vi "Checkers File Load.vi"   [LabVIEW 2016]
uses:
  Game Info Global Variable.vi
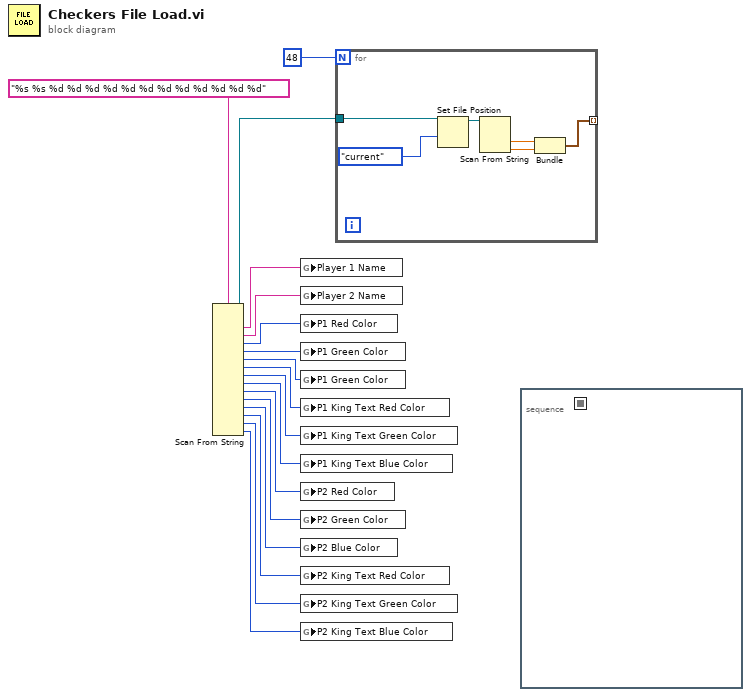
[diagram p0: block diagram]
diagram:
  n1 = Scan From String("%s %s %d %d %d %d %d %d %d %d %d %d %d %d" ("format string")) -> (w16:refnum<file>, output 1=w14:string, output 2=w13:string, output 3=w12:i32, output 4=w11:i32, output 5=w10:i32, output 6=w9:i32, output 7=w8:i32, output 8=w7:i32, output 9=w6:i32, output 10=w5:i32, output 11=w4:i32, output 12=w3:i32, output 13=w2:i32, output 14=w1:i32)  [unwired: 16 in, 1 out]
  n2 = global write "Game Info Global Variable.vi" "Player 1 Name"(w14) -> ()
  n3 = global write "Game Info Global Variable.vi" "Player 2 Name"(w13) -> ()
  n4 = global write "Game Info Global Variable.vi" "P1 Red Color"(w12) -> ()
  n5 = global write "Game Info Global Variable.vi" "P1 Green Color"(w11) -> ()
  n6 = global write "Game Info Global Variable.vi" "P1 Green Color"(w10) -> ()
  n7 = global write "Game Info Global Variable.vi" "P1 King Text Red Color"(w9) -> ()
  n8 = global write "Game Info Global Variable.vi" "P1 King Text Green Color"(w8) -> ()
  n9 = global write "Game Info Global Variable.vi" "P1 King Text Blue Color"(w7) -> ()
  n10 = global write "Game Info Global Variable.vi" "P2 Red Color"(w6) -> ()
  n11 = global write "Game Info Global Variable.vi" "P2 Green Color"(w5) -> ()
  n12 = global write "Game Info Global Variable.vi" "P2 Blue Color"(w4) -> ()
  n13 = global write "Game Info Global Variable.vi" "P2 King Text Red Color"(w3) -> ()
  n14 = global write "Game Info Global Variable.vi" "P2 King Text Green Color"(w2) -> ()
  n15 = global write "Game Info Global Variable.vi" "P2 King Text Blue Color"(w1) -> ()
  n16 = for {
    N: 48 -> [_]
    tunnel: [w21] -> _ mode=indexing
    tunnel: w16 -> [w19]
    n17 = Set File Position(refnum=w19, from (0:start)=enum16{"start", "end", "current"}."current") -> (refnum out=w18:refnum<file>)  [unwired: 2 in, 1 out]
    n18 = Scan From String(w18) -> (output 1=w23:dbl, output 2=w22:dbl)  [unwired: 4 in, 2 out]
    n19 = Bundle(w23, w22) -> (w21:cluster{dbl, dbl})  [unwired: 1 in]
  }
  n20 = stacked-sequence {
    frame #0 {
    }
  }
